vi "COMConfigure.vi"(6 "COMResponsiveness":T1, 8 "ErrorIn":errorcluster, 10 "COMConfig":T2={"BaudRate"=9600, "DataBits"=8, "Parity"=enum."None", "StopBits"=10, "DataTransferTimeout[ms]"=1000, "FastTransferTimeout[ms]"=100, "ConnTries"=0, "MsWaitBeforeRetry"=0} {"StopBits" items=["1.0"=10, "1.5"=15, "2.0"=20]; "DataBits" min=7 max=9 step=1; "BaudRate" min=9600 max=921600 step=1}, 11 "COMHandlerIn":refnum<visa-resource-name>) -> (0 "ErrorOut":errorcluster, 3 "COMHandlerOut":refnum<visa-resource-name>)   [LabVIEW 2016]
doc: "Configure COM port for the application's purpose.\n\nApplication implements timeouts for operations (COMResponsiveness):\n- fast transfer,\n- data transfer.\n\nCOMConfig structure provides all available information which could change during application running. However, you need to reopen serial port in order to properly change communication port parameters. This VI requires opened serial port!"
uses:
  COMConfig.ctl
  COMResponsiveness.ctl
  <vilib>/Instr/_visa.llb/VISA Configure Serial Port (Instr).vi
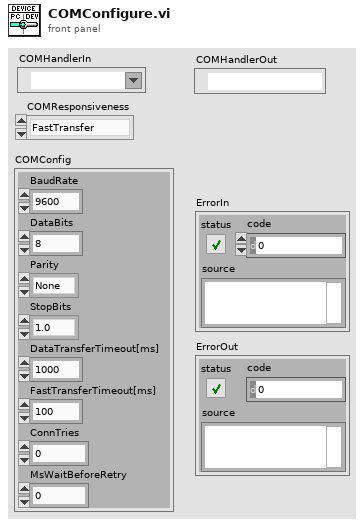
[diagram p1: front panel]
types:
  T1 = typedef "COMResponsiveness.ctl" = enum16{"FastTransfer", "DataTransfer"}
  T2 = typedef "COMConfig.ctl" = cluster{"BaudRate":u32, "DataBits":u16, "Parity":enum16{"None", "Odd", "Even", "Mark", "Space"}, "StopBits":u16, "DataTransferTimeout[ms]":u32, "FastTransferTimeout[ms]":u32, "ConnTries":i32, "MsWaitBeforeRetry":u32}
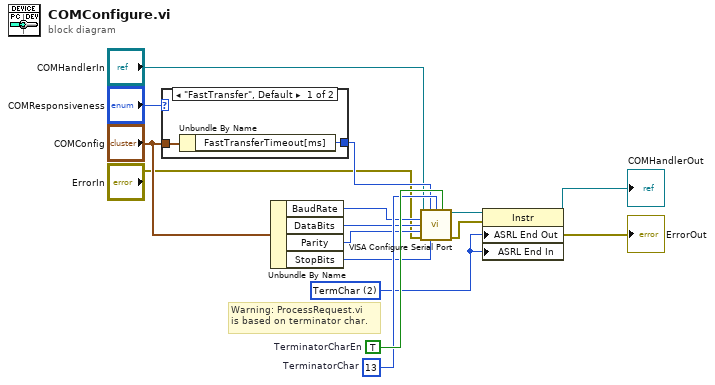
[diagram p0: block diagram]
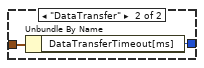
[diagram p2: hidden frame]
diagram:
  w1 = u16 2 items=["None", "Last Bit", "TermChar", "Break"] ("Serial Settings:End Mode for Writes")
  w16 = TRUE  # TerminatorCharEn
  w15 = u8 13  # TerminatorChar
  # "Warning: ProcessRequest.vi \nis based on terminator char."
  n1 = case shown="\"FastTransfer\", Default" "COMResponsiveness" {
    tunnel: "COMConfig" -> [w18 w20]
    tunnel: [w17 w19] -> w8
    frame "FastTransfer", Default {
      n2 = Unbundle By Name(w18) -> ("FastTransferTimeout[ms]"=w17:u32)
    }
    frame "DataTransfer" {
      n3 = Unbundle By Name(w20) -> ("DataTransferTimeout[ms]"=w19:u32)
    }
  }
  n4 = Unbundle By Name("COMConfig") -> ("BaudRate"=w12:u32, "DataBits"=w11:u16, "Parity"=w10:enum16{"None", "Odd", "Even", "Mark", "Space"}, "StopBits"=w9:u16)
  n5 = call-poly "VISA Configure Serial Port"("VISA resource name"="COMHandlerIn", "timeout (10sec)"=w8, "termination char\n(0xA = '\\n' = LF)"=w15, "Enable Termination\nChar (T)"=w16, "baud rate (9600)"=w12, "data bits (8)"=w11, "parity (0:none)"=w10, "error in (no error)"="ErrorIn", "stop bits (10: 1 bit)"=w9) -> ("VISA resource name out"=w5:refnum<visa-resource-name>, "error out"=w4:errorcluster)  [unwired: 5 in]
  n6 = property class="Instr"(reference=w5, error in=w4, "ASRL End Out"=w1, "ASRL End In"=w1) -> (reference out=→"COMHandlerOut":refnum<visa-resource-name>, error out=→"ErrorOut":errorcluster)
